vi "Odometria.vi"(6 "d":dbl, 9 "Zigma":dbl[](array[numeric]), 10 "right motor ccw velocity (rad/s)":dbl, 11 "left motor ccw velocity (rad/s)":dbl) -> (3 "Intregral":dbl[](array[numeric]))   [LabVIEW 2011]
panel:
  out "Arrastrado 2":dbl[](array[numeric])
  in  "Arrastrado":dbl[](array[numeric])
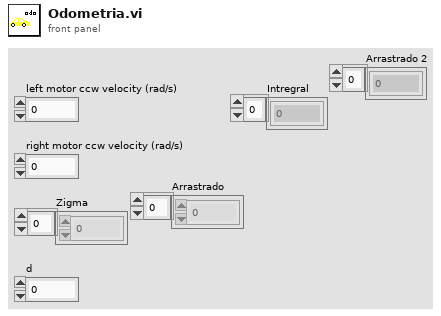
[diagram p1: front panel]
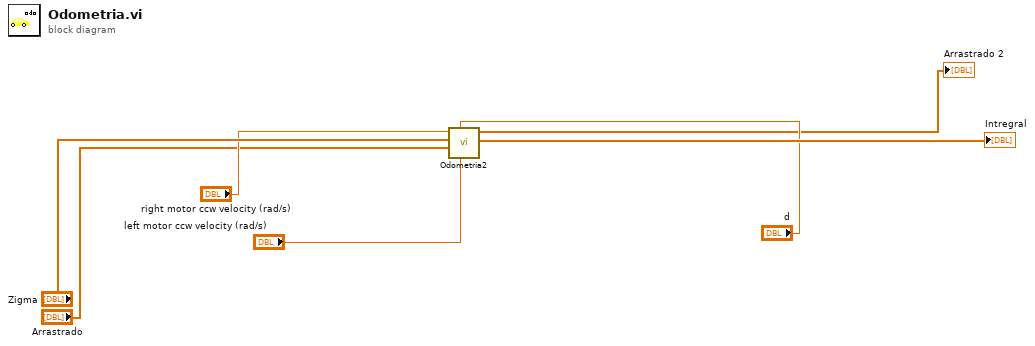
[diagram p0: block diagram]
diagram:
  n1 = call "Odometria2.vi"("left motor ccw velocity (rad/s)"="left motor ccw velocity (rad/s)", "d"="d", "Arrastrado"="Arrastrado", "Zigma"="Zigma", "right motor ccw velocity (rad/s)"="right motor ccw velocity (rad/s)") -> ("Array out"=→"Intregral":dbl[], "A x Vector"=→"Arrastrado 2":dbl[])  [unwired: 5 in]
